vi "LVPortProcessMatlabEvents.vi"(8 "error in":errorcluster, 11 "pID":string) -> (0 "error out":errorcluster)   [LabVIEW 2017]
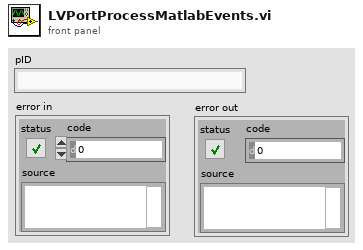
[diagram p1: front panel]
types:
  T1 = typedef "LVPortEventRegistrationDataType.ctl" = refnum<event-registration>
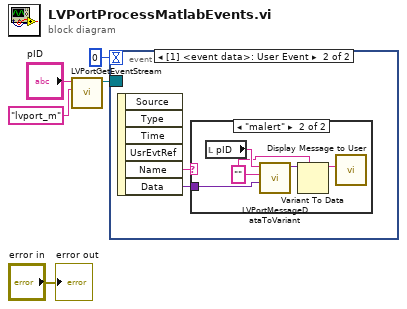
[diagram p0: block diagram]
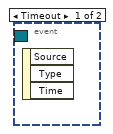
[diagram p2: hidden frame]
diagram:
  n1 = call "LVPortGetEventStream.vi"("Category"="lvport_m", "ID"="pID") -> ("Event Registration Refnum out"=w3:T1)  [unwired: 6 in, 3 out]
  n2 = event shown="[1] <event data>: User Event" {
    selector: w3 -> [_ _]
    dyn-events: _ -> [_ _]
    timeout: 0 -> [_ _]
    event Timeout {
      n3 = event-data() -> ()  [unwired: 1 in, 3 out]
    }
    event User Event {
      n4 = event-data() -> ("Name"=w7:string, "Data"=w6:variant)  [unwired: 1 in, 4 out]
      n5 = case shown="\"malert\"" w7 {
        tunnel: w6 -> [_ w9]
        frame "False", Default {
        }
        frame "malert" {
          w8 = ""
          n6 = local read "pID"() -> (w12:string)
          n7 = call "LVPortMessageDataToVariant.vi"("Message Data Object"=w9, "Value type (or value to update)"=w8, "pID"=w12) -> ("Value"=w11:variant)  [unwired: 8 in]
          n8 = Variant To Data(type=w8, Variant=w11) -> (data=w10:string)  [unwired: 1 in, 1 out]
          n9 = call "Display Message to User"("Message"=w10) -> ()  [unwired: 9 in, 2 out]
        }
      }
    }
  }
  "error out" <- "error in"
